vi "Online Filtering - DFD.vi"() -> ()   [LabVIEW 2023]
doc: "Uses VIs in the LabVIEW Digital Filter Design Toolkit to perform online filtering without having to compensate for the initial transient after the first block of data is filtered. This example repeatedly generates a noisy sine wave and filters it using two different methods.\n\nThe first method uses the memory mechanism to retain state information about the previous filtering process to eliminate the transient. \n\nThe second method uses no memory mechanism and assumes zero initial states each time the VI is called. The result is that this method produces a transient on each iteration rather than the filtered signal."
uses:
  <vilib>/addons/Digital Filter Design/Process.llb/DFD Filtering (Array).vi
  <vilib>/Analysis/NI_AALBase.lvlib
  <vilib>/addons/Digital Filter Design/NI_DigFilterLicensed.lvlib
panel:
  out "Filtered Signal using\nSingle Mode":dbl[](graph)
  in  "# points":i32=31
  in  "stop":bool
  out "Filtered Signal using\nContinuous Mode":dbl[](graph)
  out "Original Noisy Signal":dbl[](graph)
  # "Notice that the initial transient\nexists only for the first call to the\nIIR Cascade Filter VI."
  # "Notice that the initial transient exists \neverytime the IIR Cascade Filter VI is \ncalled causing significant distortion."
  # "Select Help»Show Context Help and move the cursor over the VI icon for more information."
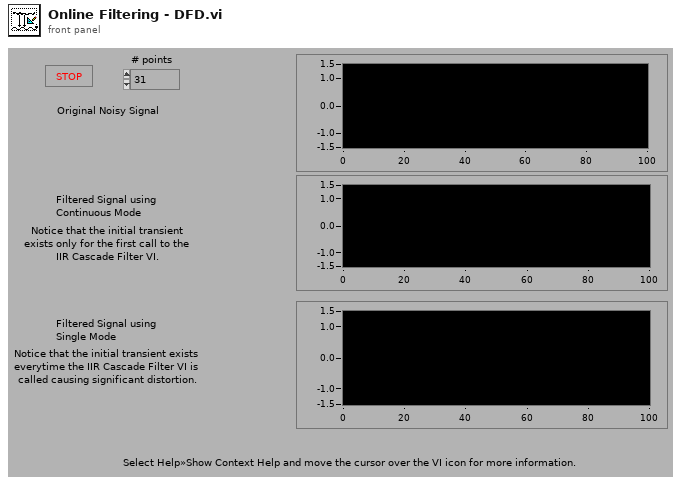
[diagram p1: front panel]
types:
  T1 = enum16{"Lowpass", "Highpass", "Bandpass", "Bandstop"}
  T2 = typedef "NI_DigFilterLicensed.lvlib/DFD Filter Obj.ctl" = cluster{"mSRate_Fs":dbl, "mSRate_Version":string, "mSRate_Comments":string, "mSRate_OrgCoef":T3, "mSRate_CurCoef":T3, "mSRate_Quantized?":bool, "mSRate_QCoef":T3, "mSRate_QSettings":T5[], "mSRate_Order":i32, "mSRate_Scaling":cluster{"mSRate_ScaleByPowerOf2?":bool, "mSRate_ScaleType":T7}}
  T3 = typedef "NI_DigFilterLicensed.lvlib/DFD Filter Coef.ctl" = cluster{"type":T4, "gain":dbl, "coef a (k)":dbl[], "coef b (v)":dbl[]}
  T4 = typedef "NI_DigFilterLicensed.lvlib/DFD Filter Structure Type Selector.ctl" = enum16{"Undefined", "FIR Direct Form", "FIR Direct Form Transposed", "FIR Symmetric", "FIR Antisymmetric", "IIR Direct Form I", "IIR Direct Form I Transposed", "IIR Direct Form II", "IIR Direct Form II Transposed", "IIR Cascaded Second Order Sections Form I", "IIR Cascaded Second Order Sections Form I Transposed", "IIR Cascaded Second Order Sections Form II", "IIR Cascaded Second Order Sections Form II Transposed", "Lattice Allpass (basic sections)", "Lattice Allpass (one multiplier sections)", "Lattice Allpass (normalized sections)", "Lattice AR (basic sections)", "Lattice AR (one multiplier sections)", "Lattice AR (normalized sections)", "Lattice MA (minimum phase)", "Lattice MA (maximum phase)", "Lattice ARMA (basic sections)", "Lattice ARMA (one multiplier sections)", "Lattice ARMA (normalized sections)"}
  T5 = typedef "NI_DigFilterLicensed.lvlib/dfd_Internal Quantization Settings.ctl" = cluster{"source":T6, "wl":i16, "iwl":i16, "overflow mode":enum16{"Saturation", "Wrap"}, "rounding mode":enum16{"Nearest", "Truncation"}, "signed?":bool}
  T6 = typedef "NI_DigFilterLicensed.lvlib/dfd_Internal Quantization Srcs.ctl" = u16
  T7 = typedef "NI_DigFilterLicensed.lvlib/DFD Coef Norm Type.ctl" = enum16{"No Norm", "Time Domain 1-Norm", "Time Domain 2-Norm", "Time Domain Inf-Norm"}
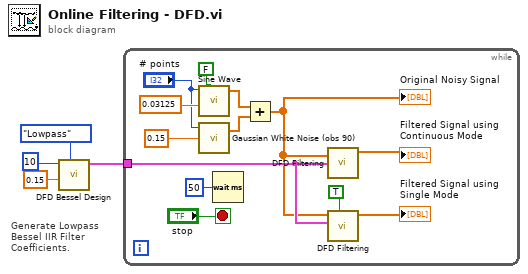
[diagram p0: block diagram]
diagram:
  # "Generate Lowpass\nBessel IIR Filter \nCoefficients."
  n1 = call <vilib>:"DFD Bessel Design.vi"("filter type"=T1."Lowpass", "low cutoff freq [Hz]"=0.15, "order"=10) -> ("filter out"=w4:T2)  [unwired: 3 in, 5 out]
  n2 = while {
    tunnel: w4 -> [w12]
    stop <- "stop" stop-if-true
    n3 = call <vilib>:"Sine Wave.vi"("samples"="# points", "frequency"=0.03125, "reset phase"=FALSE) -> ("sine wave"=w11:dbl[])  [unwired: 2 in, 2 out]
    n4 = call <vilib>:"Gaussian White Noise (obs 90).vi"("standard deviation"=0.15, "samples"="# points") -> ("Gaussian noise pattern"=w16:dbl[])  [unwired: 1 in, 1 out]
    n5 = Wait (ms)(milliseconds to wait=u32 50) -> ()  [unwired: 1 out]
    n6 = Add(x=w11, y=w16) -> (x+y=w10:dbl[])
    "Original Noisy Signal" <- w10
    n7 = call-poly <vilib>:"DFD Filtering.vi"("filter"=w12, "signal in"=w10) -> ("signal out"=→"Filtered Signal using\nContinuous Mode":dbl[])  [unwired: 2 in, 7 out]
    n8 = call-poly <vilib>:"DFD Filtering.vi"("init? (F)"=TRUE, "filter"=w12, "signal in"=w10) -> ("signal out"=→"Filtered Signal using\nSingle Mode":dbl[])  [unwired: 1 in, 7 out]
  }
